vi "SEH Sort and Convert Ranges.vi"(8 "error in (no error)":errorcluster, 10 "Error Display Options":T3[](array[typedef])) -> (0 "error out":errorcluster, 1 "Detect Any Warnings":bool, 2 "Error Processing Options":T2[](array[typedef]), 4 "Valid Default":bool, 6 "Default Action":T1={"Number of Retries"=0, "Output Classification"="*Non-critical*", "Retry"=FALSE, "Classify Output"=FALSE, "Classify Notification"=FALSE, "Notification Classification"="*Non-critical*", "Convert Output to Warning"=FALSE, "Clear Output"=FALSE, "Notify"=FALSE, "Priority"=0, "Detect Warning"=FALSE, "Call VI"=FALSE, "VI to Call"="*Non-critical*"})   [LabVIEW 2014]
uses:
  Controls/SEH/SEH Error Display Options.ctl
  Controls/SEH/SEH Shared Error Options.ctl
  Controls/SEH/SEH Error Options.ctl
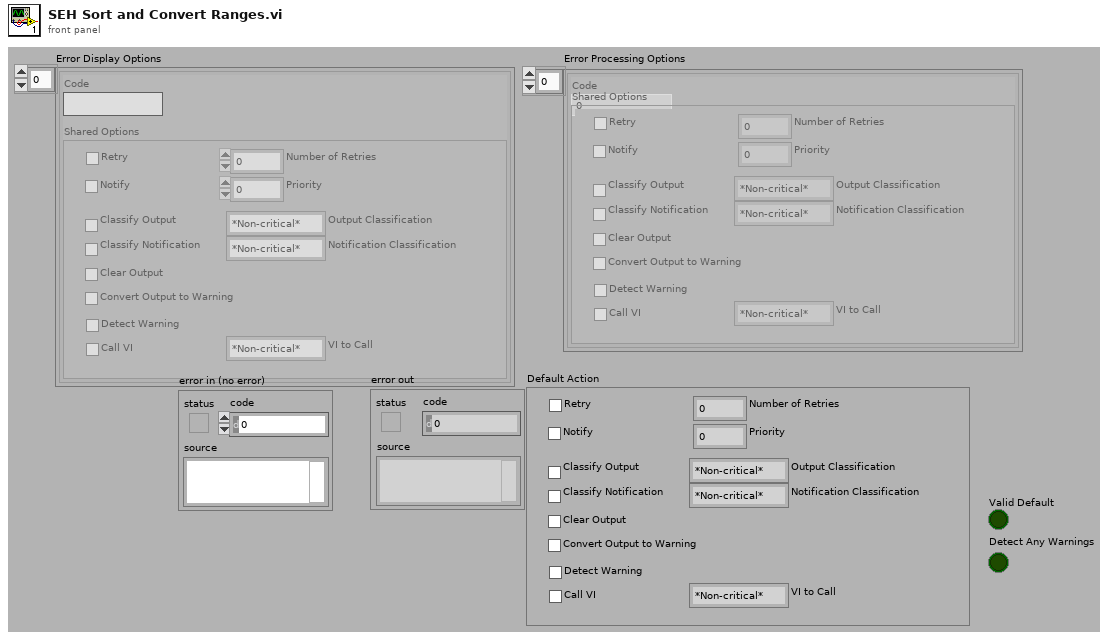
[diagram p1: front panel]
types:
  T1 = typedef "SEH Shared Error Options.ctl" = cluster{"Number of Retries":i32, "Output Classification":string, "Retry":bool, "Classify Output":bool, "Classify Notification":bool, "Notification Classification":string, "Convert Output to Warning":bool, "Clear Output":bool, "Notify":bool, "Priority":i32, "Detect Warning":bool, "Call VI":bool, "VI to Call":string}
  T2 = typedef "SEH Error Options.ctl" = cluster{"Code":i32, "Shared Options":T1}
  T3 = typedef "SEH Error Display Options.ctl" = cluster{"Code":string, "Shared Options":T1}
  T4 = typedef "SEH Code Types.ctl" = enum16{"Code", "Range", "Category", "Invalid", "Default Action"}
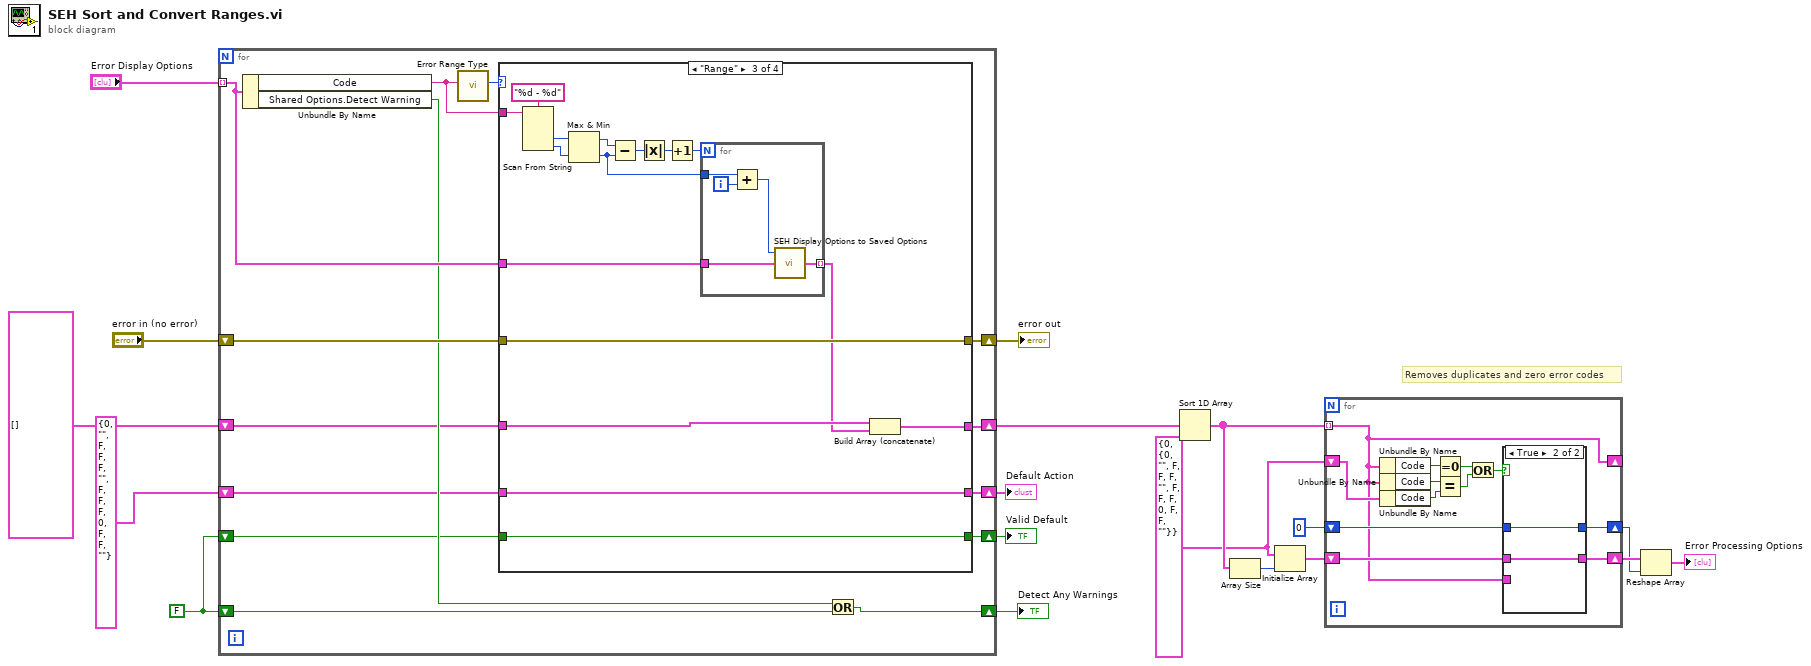
[diagram p0: block diagram]
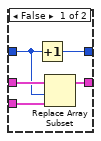
[diagram p2: hidden frame]
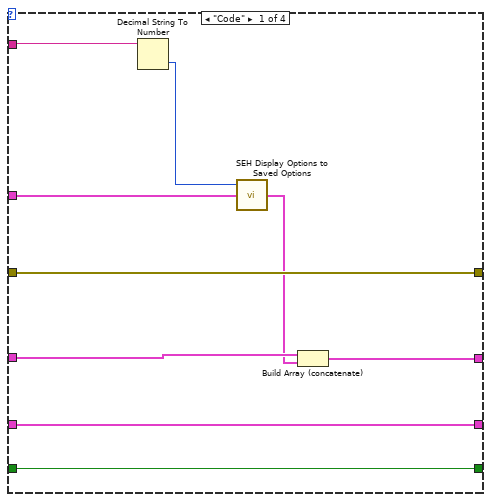
[diagram p3: hidden frame]
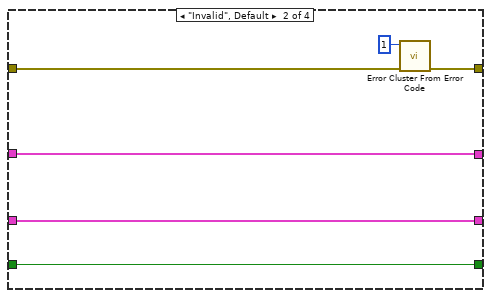
[diagram p4: hidden frame]
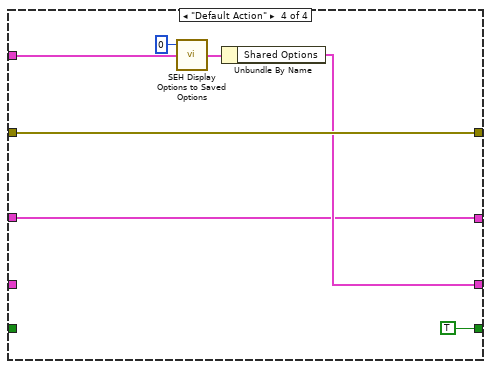
[diagram p5: hidden frame]
diagram:
  w3 = FALSE
  w15 = T2 {"Code"=0, "Shared Options"={"Number of Retries"=0, "Output Classification"="", "Retry"=FALSE, "Classify Output"=FALSE, "Classify Notification"=FALSE, "Notification Classification"="", "Convert Output to Warning"=FALSE, "Clear Output"=FALSE, "Notify"=FALSE, "Priority"=0, "Detect Warning"=FALSE, "Call VI"=FALSE, "VI to Call"=""}} ("Error Options")
  # "Removes duplicates and zero error codes"
  n1 = for {
    tunnel: "Error Display Options" -> [w30] mode=indexing
    shift-right: [w28] -> w8
    shift-left: "error in (no error)" -> [w29]
    shift-right: [w25] -> w7
    shift-left: w3 -> [w26]
    shift-right: [w23] -> w5
    shift-left: T2[] [] -> [w24]
    shift-right: [w20] -> w2
    shift-left: T1 {"Number of Retries"=0, "Output Classification"="", "Retry"=FALSE, "Classify Output"=FALSE, "Classify Notification"=FALSE, "Notification Classification"="", "Convert Output to Warning"=FALSE, "Clear Output"=FALSE, "Notify"=FALSE, "Priority"=0, "Detect Warning"=FALSE, "Call VI"=FALSE, "VI to Call"=""} ("Shared Options") -> [w21]
    shift-right: [w19] -> w1
    shift-left: w3 -> [w22]
    n2 = Unbundle By Name(w30) -> ("Code"=w31:string, "Shared Options.Detect Warning"=w27:bool)
    n3 = call "Error Range Type.vi"("Codes"=w31) -> ("Type"=w32:T4)  [unwired: 10 out]
    n4 = case shown="\"Range\"" w32 {
      tunnel: w31 -> [w41 _ w63 _]
      tunnel: w30 -> [w38 _ w58 w75]
      tunnel: w29 -> [w40 w47 w53 w73]
      tunnel: [w40 w46 w53 w73] -> w28
      tunnel: w24 -> [w37 w44 w52 w70]
      tunnel: [w35 w44 w50 w70] -> w23
      tunnel: w22 -> [w33 w42 w49 _]
      tunnel: w21 -> [w34 w43 w48 _]
      tunnel: [w34 w43 w48 w71] -> w20
      tunnel: [w33 w42 w49 TRUE] -> w19
      frame "Code" {
        n5 = Decimal String To Number(string=w41) -> (number=w39:i32)  [unwired: 3 out]
        n6 = call "SEH Display Options to Saved Options.vi"("Display Error Options"=w38, "Code"=w39) -> ("Saved Error Options"=w36:T2)  [unwired: 1 in]
        n7 = Build Array (concatenate)(w37, w36) -> (w35:T2[])
      }
      frame "Invalid", Default {
        n8 = call <vilib>:"Error Cluster From Error Code.vi"("error in (no error)"=w47, "error code (0)"=1) -> ("error out"=w46:errorcluster)  [unwired: 1 in, 6 out]
      }
      frame "Range" {
        n9 = Scan From String(format string="%d - %d", input string=w63) -> (output 1=w61:i32, output 2=w60:i32)  [unwired: 2 in, 5 out]
        n10 = Max & Min(x=w61, y=w60) -> (max(x,y)=w57:i32, min(x,y)=w56:i32)
        n11 = Subtract(x=w57, y=w56) -> (x-y=w59:i32)
        n12 = Absolute Value(x=w59) -> (abs(x)=w55:i32)
        n13 = Increment(x=w55) -> (x+1=w54:i32)
        n14 = for {
          N: w54 -> [_]
          tunnel: w58 -> [w64]
          tunnel: w56 -> [w68]
          tunnel: [w65] -> w51 mode=indexing
          i -> [w67]
          n15 = Add(x=w68, y=w67) -> (x+y=w66:i32)
          n16 = call "SEH Display Options to Saved Options.vi"("Display Error Options"=w64, "Code"=w66) -> ("Saved Error Options"=w65:T2)  [unwired: 1 in]
        }
        n17 = Build Array (concatenate)(w52, w51) -> (w50:T2[])
      }
      frame "Default Action" {
        n18 = call "SEH Display Options to Saved Options.vi"("Display Error Options"=w75, "Code"=0) -> ("Saved Error Options"=w72:T2)  [unwired: 1 in]
        n19 = Unbundle By Name(w72) -> ("Shared Options"=w71:T1)
      }
    }
    n20 = Or(x=w27, y=w26) -> (x .or. y?=w25:bool)
  }
  "error out" <- w8
  "Detect Any Warnings" <- w7
  "Default Action" <- w2
  "Valid Default" <- w1
  n21 = Sort 1D Array(array=w5) -> (sorted array=w16:T2[])
  n22 = Array Size(array=w16) -> (size(s)=w14:i32)
  n23 = Initialize Array(w15, w14) -> (w13:T2[])
  n24 = for {
    tunnel: w16 -> [w76] mode=indexing
    shift-right: [w76] -> _
    shift-left: w15 -> [w85]
    shift-right: [w79] -> w11
    shift-left: 0 -> [w80]
    shift-right: [w77] -> w12
    shift-left: w13 -> [w78]
    n25 = Unbundle By Name(w76) -> ("Code"=w84:i32)
    n26 = Unbundle By Name(w76) -> ("Code"=w87:i32)
    n27 = Unbundle By Name(w85) -> ("Code"=w86:i32)
    n28 = Equal To 0?(x=w84) -> (x = 0?=w83:bool)
    n29 = Equal?(x=w87, y=w86) -> (x = y?=w82:bool)
    n30 = Or(x=w83, y=w82) -> (x .or. y?=w81:bool)
    n31 = case shown="True" w81 {
      tunnel: w80 -> [w89 w93]
      tunnel: [w92 w93] -> w79
      tunnel: w78 -> [w91 w94]
      tunnel: [w90 w94] -> w77
      tunnel: w76 -> [w88 _]
      frame False {
        n32 = Increment(x=w89) -> (x+1=w92:i32)
        n33 = Replace Array Subset(array=w91, new element=w88, index=w89) -> (w90:T2[])
      }
      frame True {
      }
    }
  }
  n34 = Reshape Array(w12, w11) -> (→"Error Processing Options":T2[])
